vi "HV_Manual_Control.vi"(5 "Channel                            Voltage (V)                      Current Max (uA)             On/Off":string[][](array[string])=[["0", "1500", "100", "Off"], ["1", "1500", "100", "Off"], ["2", "1500", "100", "Off"], ["3", "1500", "100", "Off"], ["4", "1500", "100", "Off"], ["5", "1500", "100", "Off"], ["6", "1500", "100", "Off"], ["7", "1500", "100", "Off"], ["8", "1500", "100", "Off"], ["9", "1500", "100", "Off"], ["10", "1500", "100", "Off"], ["11", "1500", "100", "Off"], ["12", "1500", "100", "Off"], ["13", "1500", "100", "Off"], ["14", "1500", "100", "Off"], ["15", "1500", "100", "Off"], ["16", "1500", "100", "Off"], ["17", "1500", "100", "Off"]], 6 "Ramp Rate (V/s)":string="100", 7 "Ramp Up/Down":enum16{"Ramp Down", "Ramp Up"}(ring)=enum."Ramp Up", 10 "Parameter":T2(ring), 11 "Apply":bool) -> (3 "?":T3={"Volt Monitor"=[["", "", "", "", "", "", "", "", ""], ["", "", "", "", "", "", "", "", ""], ["", "", "", "", "", "", "", "", ""], ["", "", "", "", "", "", "", "", ""], ["", "", "", "", "", "", "", "", ""], ["", "", "", "", "", "", "", "", ""], ["", "", "", "", "", "", "", "", ""], ["", "", "", "", "", "", "", "", ""], ["", "", "", "", "", "", "", "", ""], ["", "", "", "", "", "", "", "", ""], ["", "", "", "", "", "", "", "", ""], ["", "", "", "", "", "", "", "", ""], ["", "", "", "", "", "", "", "", ""]], "On/Off"=[FALSE, FALSE, FALSE, FALSE, FALSE, FALSE, FALSE, FALSE, FALSE, FALSE, FALSE, FALSE], "Rampup"=[FALSE, FALSE, FALSE, FALSE, FALSE, FALSE, FALSE, FALSE, FALSE, FALSE, FALSE, FALSE], "Rampdown"=[FALSE, FALSE, FALSE, FALSE, FALSE, FALSE, FALSE, FALSE, FALSE, FALSE, FALSE, FALSE], "Status Errors"=["            ", "            ", "            ", "            ", "            ", "            ", "            ", "            ", "            ", "            ", "            ", "            "], "sethv Errors (Err: 0 = no error):\nVolt monitor      Status"=[]})   [LabVIEW 2018]
panel:
  in  "Close":bool
  in  "Off":bool
  in  "?":T1(tab)=enum."Timer"
  in  "Max Voltage":string="100"
  in  "Channel                            On/Off":string[][](array[string])=[["0", "Off", "100", "Off"], ["1", "Off", "100", "Off"], ["2", "Off", "100", "Off"], ["3", "Off", "100", "Off"], ["4", "Off", "100", "Off"], ["5", "Off", "100", "Off"], ["6", "Off", "100", "Off"], ["7", "Off", "100", "Off"], ["8", "Off", "100", "Off"], ["9", "Off", "100", "Off"], ["10", "Off", "100", "Off"], ["11", "Off", "100", "Off"], ["12", "Off", "100", "Off"], ["13", "Off", "100", "Off"], ["14", "Off", "100", "Off"], ["15", "Off", "100", "Off"], ["16", "Off", "100", "Off"], ["17", "Off", "100", "Off"]]
  in  "Time (s)":u32=20
  in  "Timer":bool
  out "Time Elapsed":u32
  out "Run Completed":bool
  # "Use this table to enter values.\nPlease see the monitor tab to see\ncurrent settings of HV cards."
  # "Turning all channels off at once:\nPress the \"OFF\" button\n\nVMax:\nChoose VMax parameter\nEnter maximum software voltage (up to 6000V)\nPress Apply button\n\nRampSet:\nChoose RampSet parameter\nSelect whether to set ramp up or ramp down rate\nEnter Ramp Rate in V/s\nPress Apply button\n\nMonitor:\nThe status of the channels is constantly monitored in the background in the Monitor tab if the program is running\n\nStop the program using the \"CLOSE\" button. This closes the vi and ramp all channels down."
  # "Inputting data into table:\nIn the Controls panel, there is a table to allow the channels, voltage, current and on/off state to be entered.\nEach row will correspond to the channel entered into that row.\nThis allows any channels to be used and allows the order to be changed.\nThis table does not display the current settings, it is only used to enter values\n\nVSet:\nSelect VSet parameter\nInput the voltages (V) in the Voltage column of the table in the Controls panel\nThe voltage will be for the channel selected in the same row\nPress Apply button\n\nISet:\nSelect ISet parameter\nInput maximum current (uA) in Current column of table in the Controls panel\nThe current will be for the channel selected in the same row\nPress Apply button\n\nOn/Off:\nSelect the On/Off parameter\nEnter either 'On' or 'Off' into each cell in the table on the Controls panel\nThe on/off state will be for the channel selected in the same row\nPress Apply button"
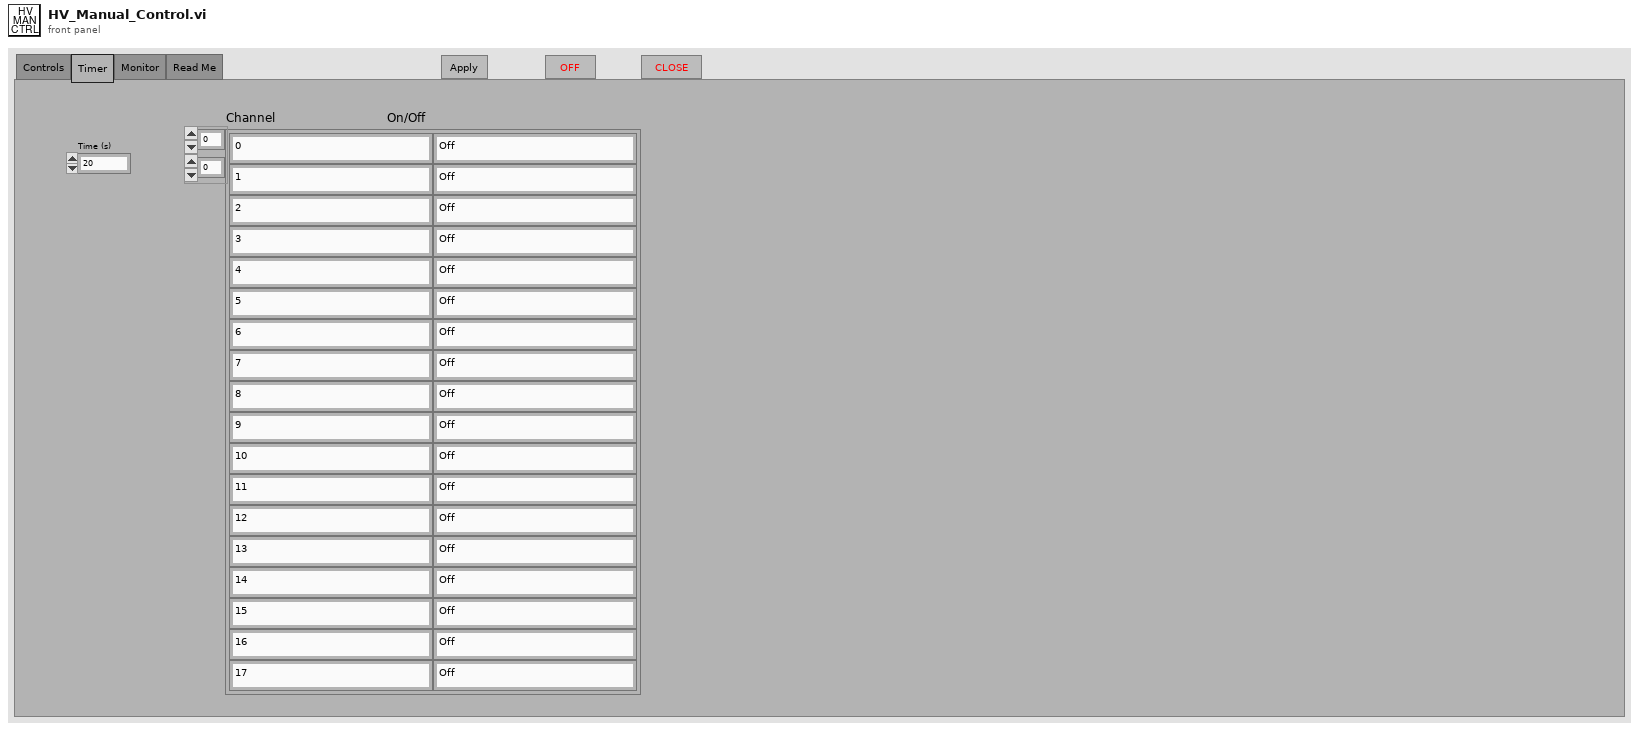
[diagram p1: front panel]
types:
  T1 = enum32{"Controls", "Timer", "Monitor", "Read Me"}
  T2 = enum16{"On/Off", "VSet", "VMax", "RampSet", "ISet"}
  T3 = cluster{"Volt Monitor":string[][], "On/Off":bool[], "Rampup":bool[], "Rampdown":bool[], "Status Errors":string[], "sethv Errors (Err: 0 = no error):\nVolt monitor      Status":string[]}
  T4 = cluster{"Volt Monitor":string[][], "On/Off":bool[], "Rampup":bool[], "Rampdown":bool[], "Status Errors":string[], "Errors:\nVolt monitor                Status":string[]}
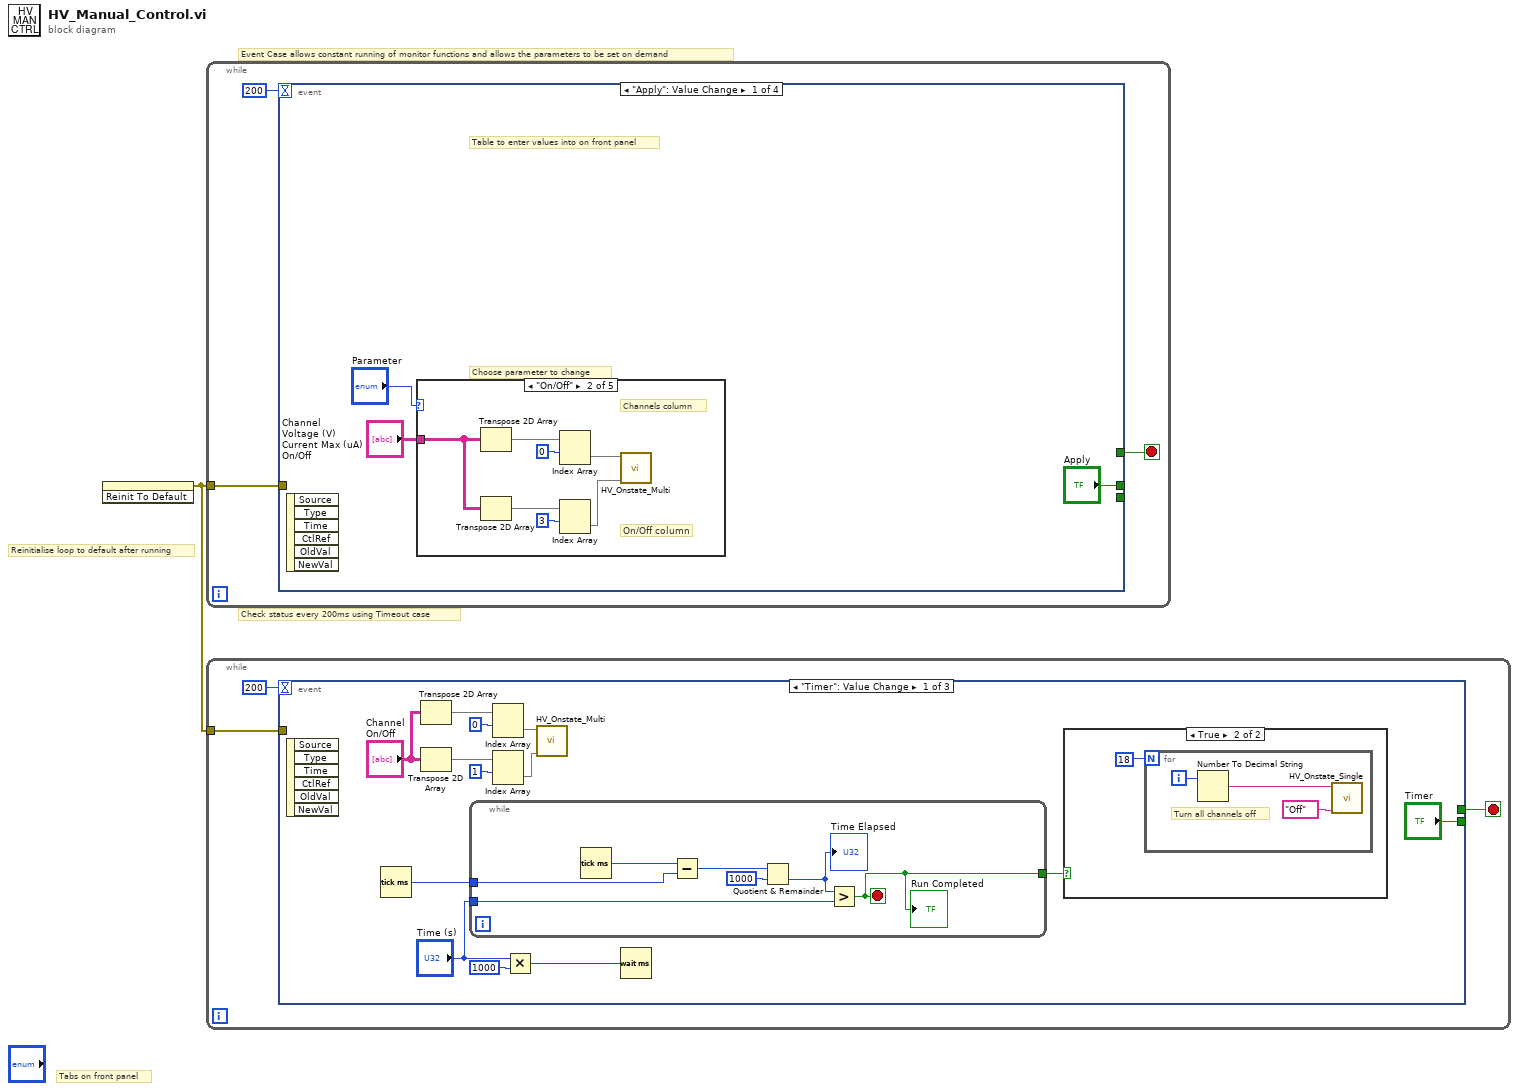
[diagram p0: block diagram]
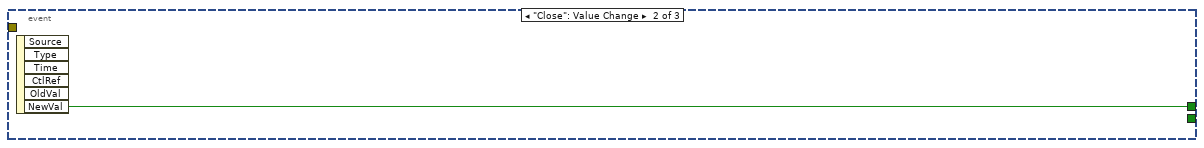
[diagram p3: hidden frame]
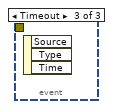
[diagram p4: hidden frame]
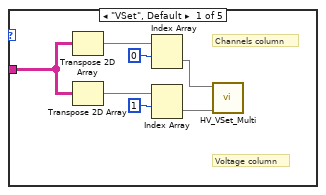
[diagram p5: hidden frame]
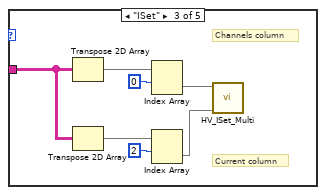
[diagram p6: hidden frame]
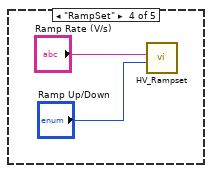
[diagram p7: hidden frame]
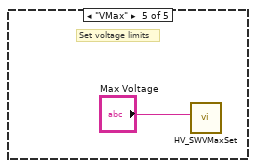
[diagram p8: hidden frame]
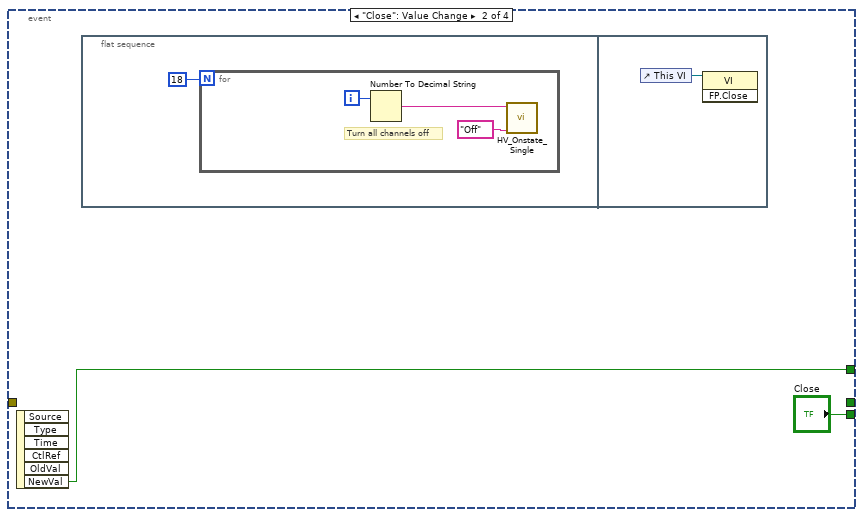
[diagram p9: hidden frame]
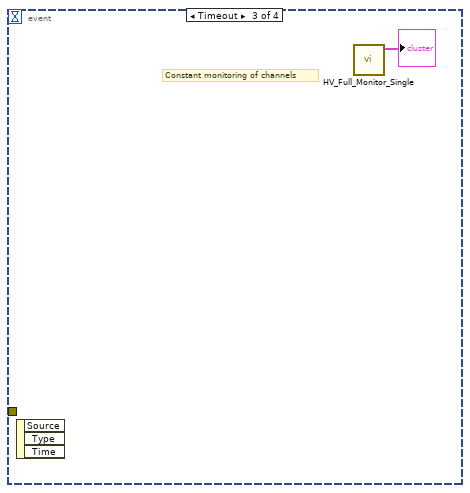
[diagram p10: hidden frame]
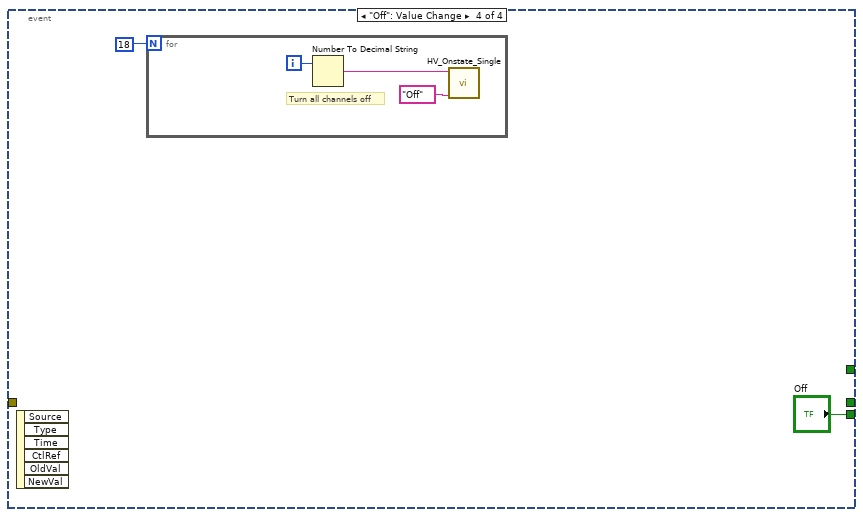
[diagram p11: hidden frame]
diagram:
  # "Check status every 200ms using Timeout case"
  # "Tabs on front panel"
  # "Reinitialise loop to default after running"
  # "Event Case allows constant running of monitor functions and allows the parameters to be set on demand"
  n1 = invoke on="Apply" class="Bool" method="Reinit To Default"() -> (error out=w1:errorcluster)  [unwired: 3 in, 2 out]
  n2 = while {
    tunnel: w1 -> [w3]
    stop <- w4 stop-if-true
    n3 = event shown="[0] \"Apply\": Value Change" {
      selector: _ -> [_ _ _ _]
      dyn-events: _ -> [_ _ _ _]
      timeout: u32 200 ("milliseconds to wait") -> [_ _ _ _]
      tunnel: [_ w32 _ _] -> w4
      tunnel: ["Apply" _ _ _] -> _
      tunnel: w3 -> [_ _ _ _]
      tunnel: [_ "Close" _ "Off"] -> _
      event "Apply": Value Change {
        # "Table to enter values into on front panel"
        # "Choose parameter to change"
        n4 = event-data() -> ()  [unwired: 1 in, 6 out]
        n5 = case shown="\"On/Off\"" "Parameter" {
          tunnel: "Channel                            Voltage (V)                      Current Max (uA)             On/Off" -> [w9 w21 w25 _ _]
          frame "VSet", Default {
            # "Voltage column"
            # "Channels column"
            n6 = Transpose 2D Array(2D array=w9) -> (transposed array=w13:string[][])
            n7 = Transpose 2D Array(2D array=w9) -> (transposed array=w10:string[][])
            n8 = Index Array(array=w13, index (row)=0) -> (element=w12:string[])  [unwired: 1 in]
            n9 = Index Array(array=w10, index (row)=1) -> (element=w8:string[])  [unwired: 1 in]
            n10 = call "HV_VSet_Multi.vi"("Voltage"=w8, "Channel"=w12) -> ()  [unwired: 9 in, 1 out]
          }
          frame "On/Off" {
            # "On/Off column"
            # "Channels column"
            n11 = Transpose 2D Array(2D array=w21) -> (transposed array=w17:string[][])
            n12 = Transpose 2D Array(2D array=w21) -> (transposed array=w18:string[][])
            n13 = Index Array(array=w17, index (row)=0) -> (element=w19:string[])  [unwired: 1 in]
            n14 = Index Array(array=w18, index (row)=3) -> (element=w20:string[])  [unwired: 1 in]
            n15 = call "HV_Onstate_Multi.vi"("On/Off"=w20, "Channel"=w19) -> ()  [unwired: 9 in, 1 out]
          }
          frame "ISet" {
            # "Current column"
            # "Channels column"
            n16 = Transpose 2D Array(2D array=w25) -> (transposed array=w28:string[][])
            n17 = Transpose 2D Array(2D array=w25) -> (transposed array=w26:string[][])
            n18 = Index Array(array=w28, index (row)=0) -> (element=w24:string[])  [unwired: 1 in]
            n19 = Index Array(array=w26, index (row)=2) -> (element=w23:string[])  [unwired: 1 in]
            n20 = call "HV_ISet_Multi.vi"("Currents"=w23, "Channels"=w24) -> ()  [unwired: 9 in, 1 out]
          }
          frame "RampSet" {
            n21 = call "HV_Rampset.vi"("Ramp Up/Down"="Ramp Up/Down", "Ramp Rate"="Ramp Rate (V/s)") -> ()  [unwired: 9 in, 1 out]
          }
          frame "VMax" {
            # "Set voltage limits"
            n22 = call "HV_SWVMaxSet.vi"("Max Voltage"="Max Voltage") -> ()  [unwired: 10 in, 1 out]
          }
        }
      }
      event "Close": Value Change {
        n23 = event-data() -> ("NewVal"=w32:bool)  [unwired: 1 in, 5 out]
        n24 = flat-sequence {
          frame #0 {
            n25 = for {
              N: 18 -> [_]
              i -> [w36]
              # "Turn all channels off"
              n26 = Number To Decimal String(number=w36) -> (decimal integer string=w37:string)  [unwired: 1 in]
              n27 = call "HV_Onstate_Single.vi"("On/Off"="Off", "Channel"=w37) -> ()  [unwired: 9 in, 1 out]
            }
          }
          frame #1 {
            n28 = control-ref of="This VI"() -> (w38:refnum<vi>)
            n29 = invoke class="VI" method="FP.Close"(reference=w38) -> ()  [unwired: 2 in, 3 out]
          }
        }
      }
      event Timeout {
        # "Constant monitoring of channels"
        n30 = event-data() -> ()  [unwired: 1 in, 3 out]
        n31 = call "HV_Full_Monitor_Single.vi"() -> ("Monitor Cluster"=→"?":T4)  [unwired: 11 in]
      }
      event "Off": Value Change {
        n32 = event-data() -> ()  [unwired: 1 in, 6 out]
        n33 = for {
          N: 18 -> [_]
          i -> [w43]
          # "Turn all channels off"
          n34 = Number To Decimal String(number=w43) -> (decimal integer string=w44:string)  [unwired: 1 in]
          n35 = call "HV_Onstate_Single.vi"("On/Off"="Off", "Channel"=w44) -> ()  [unwired: 9 in, 1 out]
        }
      }
    }
  }
  n36 = while {
    tunnel: w1 -> [w47]
    stop <- w45 stop-if-true
    n37 = event shown="[0] \"Timer\": Value Change" {
      selector: _ -> [_ _ _]
      dyn-events: _ -> [_ _ _]
      timeout: u32 200 ("milliseconds to wait") -> [_ _ _]
      tunnel: w47 -> [_ _ _]
      tunnel: [_ w72 _] -> w45
      tunnel: ["Timer" _ _] -> _
      event "Timer": Value Change {
        n38 = event-data() -> ()  [unwired: 1 in, 6 out]
        n39 = Tick Count (ms)() -> (millisecond timer value=w60:u32)
        n40 = Transpose 2D Array(2D array="Channel                            On/Off") -> (transposed array=w53:string[][])
        n41 = Transpose 2D Array(2D array="Channel                            On/Off") -> (transposed array=w54:string[][])
        n42 = while {
          tunnel: w60 -> [w66]
          tunnel: "Time (s)" -> [w63]
          tunnel: [w61] -> w57
          stop <- w61 stop-if-true
          n43 = Tick Count (ms)() -> (millisecond timer value=w67:u32)
          n44 = Subtract(x=w67, y=w66) -> (x-y=w65:u32)
          n45 = Quotient & Remainder(x=w65, y=u32 1000) -> (floor(x/y)=w62:u32)  [unwired: 1 out]
          "Time Elapsed" <- w62
          n46 = Greater?(x=w62, y=w63) -> (0:w61:bool)
          "Run Completed" <- w61
        }
        n47 = Index Array(array=w53, index (row)=0) -> (element=w55:string[])  [unwired: 1 in]
        n48 = Index Array(array=w54, index (row)=1) -> (element=w56:string[])  [unwired: 1 in]
        n49 = Multiply(x="Time (s)", y=u32 1000) -> (x*y=w58:u32)
        n50 = call "HV_Onstate_Multi.vi"("On/Off"=w56, "Channel"=w55) -> ()  [unwired: 9 in, 1 out]
        n51 = Wait (ms)(milliseconds to wait=w58) -> ()  [unwired: 1 out]
        n52 = case shown="True" w57 {
          frame False {
          }
          frame True {
            n53 = for {
              N: 18 -> [_]
              i -> [w70]
              # "Turn all channels off"
              n54 = Number To Decimal String(number=w70) -> (decimal integer string=w71:string)  [unwired: 1 in]
              n55 = call "HV_Onstate_Single.vi"("On/Off"="Off", "Channel"=w71) -> ()  [unwired: 9 in, 1 out]
            }
          }
        }
      }
      event "Close": Value Change {
        n56 = event-data() -> ("NewVal"=w72:bool)  [unwired: 1 in, 5 out]
      }
      event Timeout {
        n57 = event-data() -> ()  [unwired: 1 in, 3 out]
      }
    }
  }
